vi "FGV_all stop.vi"(7 "Enum":enum16{"Set", "Get"}(ring), 10 "All Stop":bool) -> (2 "All Stop?":bool)   [LabVIEW 2017]
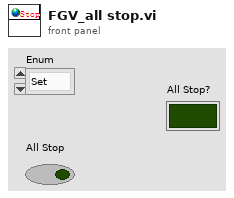
[diagram p1: front panel]
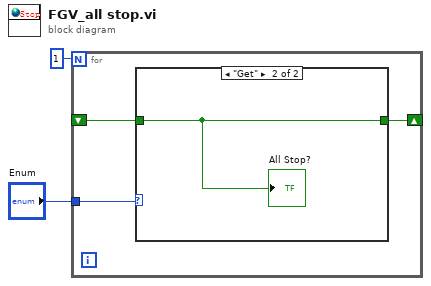
[diagram p0: block diagram]
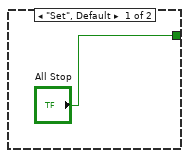
[diagram p2: hidden frame]
diagram:
  n1 = for {
    N: 1 -> [_]
    shift-right: [w4] -> _
    shift-left: _ -> [w3]
    tunnel: "Enum" -> [w5]
    n2 = case shown="\"Get\"" w5 {
      tunnel: ["All Stop" w7] -> w4
      tunnel: w3 -> [_ w7]
      frame "Set", Default {
      }
      frame "Get" {
        "All Stop?" <- w7
      }
    }
  }
